vi "PololuTicSendCommand.vi"(4 "Type":string(combo), 5 "Address":u16=16384 max=16384, 6 "Register":u8 format="%02x", 7 "Port Name":refnum<visa-resource-name>, 8 "errorIn":errorcluster, 10 "Argument":i32, 11 "PololuCommand":T2="FullScaleRatingSLPM") -> (0 "errorOut":errorcluster, 1 "LSB                                       MSB":bool[](array[boolean]) caption="Booleans", 2 "ReadValue":i64, 3 "Response":string)   [LabVIEW 2021]
uses:
  PololuCommand.ctl
  TicReplyStyle.ctl
panel:
  in  "Timeout/ms":u32=2000
  in  "ReplyType [7-bit]":T1=enum."7-bit"
  # "[16384=Unaddressed/Global]"
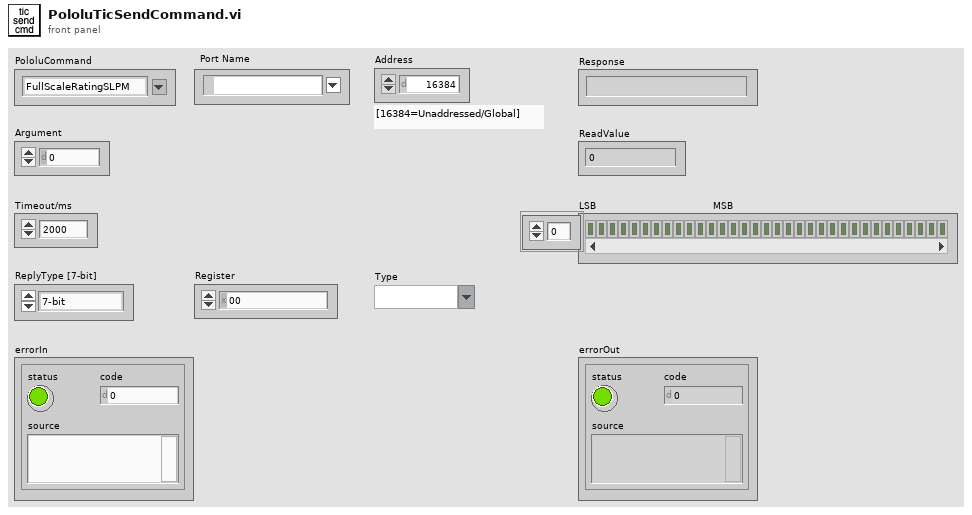
[diagram p1: front panel]
types:
  T1 = typedef "TicReplyStyle.ctl" = enum16{"8-bit", "7-bit"}
  T2 = typedef "PololuCommand.ctl" = string
  T3 = typedef "PololuCommandDescriptor.ctl" = cluster{"PololuCommand":string, "Mnemonic":string, "CommandType":T4, "Min":i32, "Max":i32}
  T4 = typedef "TicCommandType.ctl" = enum16{"Command", "7-bitWrite", "32-bitWrite", "BlockRead"}
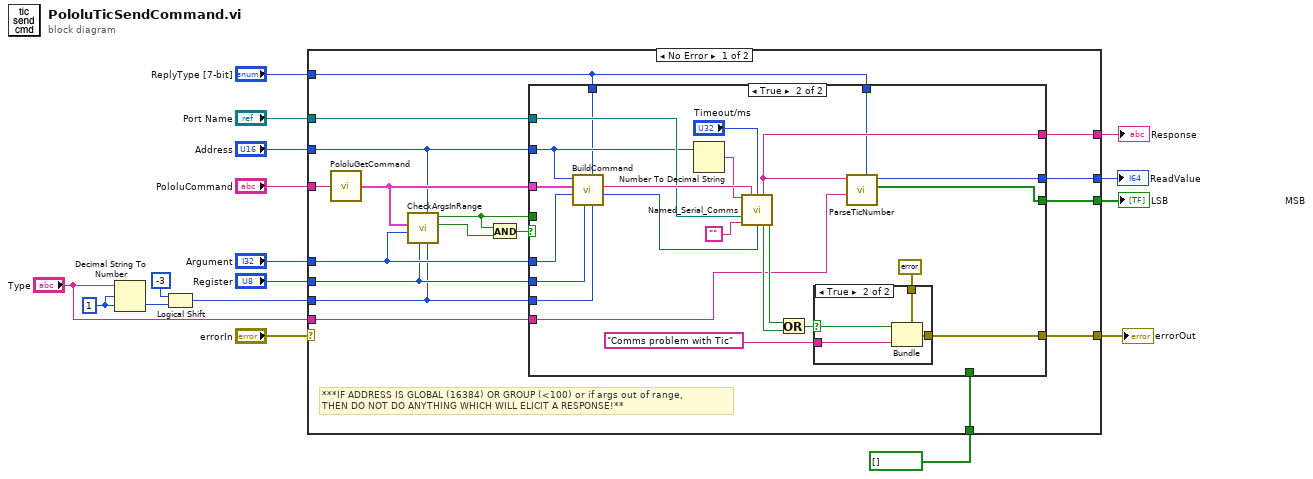
[diagram p0: block diagram]
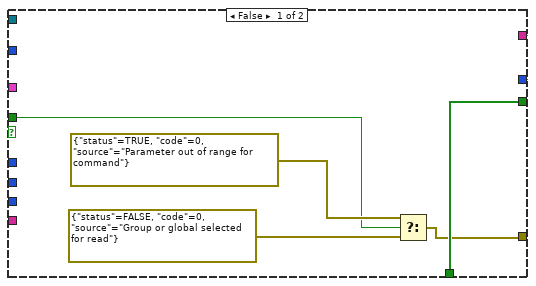
[diagram p2: hidden frame]
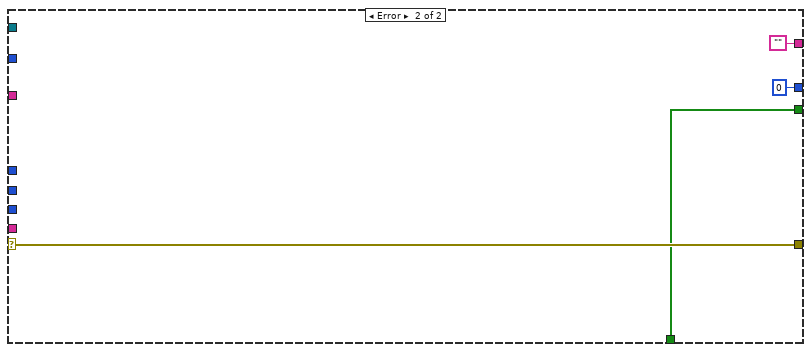
[diagram p4: hidden frame]
diagram:
  w4 = u8 1 ("offset")
  n1 = Decimal String To Number(string="Type", offset=w4, default (0L)=w4) -> (number=w7:u8)  [unwired: 1 out]
  n2 = Logical Shift(y=i16 -3, x=w7) -> (x << y=w5:u8)
  n3 = case shown="No Error" "errorIn" {
    selector: "errorIn" -> [_ w73]
    tunnel: "PololuCommand" -> [w34 _]
    tunnel: [w33 "" ("Read")] -> w16
    tunnel: [w32 i64 0 ("Value")] -> w15
    tunnel: [w31 w71] -> w14
    tunnel: [w30 w73] -> w13
    tunnel: "Argument" -> [w28 _]
    tunnel: "Register" -> [w27 _]
    tunnel: w5 -> [w26 _]
    tunnel: "Address" -> [w21 _]
    tunnel: "Port Name" -> [w25 _]
    tunnel: "Type" -> [w24 _]
    tunnel: "ReplyType [7-bit]" -> [w23 _]
    tunnel: bool[] [] ("Boolean array") -> [w22 w71]
    frame No Error {
      # "***IF ADDRESS IS GLOBAL (16384) OR GROUP (<100) or if args out of range,\nTHEN DO NOT DO ANYTHING WHICH WILL ELICIT A RESPONSE!**"
      n4 = call "PololuGetCommand.vi"("PololuCommand"=w34) -> ("CommandDescriptor"=w29:T3)  [unwired: 3 in, 1 out]
      n5 = call "CheckArgsInRange.vi"("ReadLength (bytes)"=w26, "Address"=w21, "Register"=w27, "Argument"=w28, "CommandDescriptor in"=w29) -> ("In Range?"=w19:bool, "Not Group/Global?"=w20:bool)  [unwired: 5 in]
      n6 = And(x=w20, y=w19) -> (x .and. y?=w18:bool)
      n7 = case shown="True" w18 {
        tunnel: w27 -> [_ w56]
        tunnel: w29 -> [_ w60]
        tunnel: ["" w61] -> w33
        tunnel: [0 ("Value") w64] -> w32
        tunnel: w26 -> [_ w46]
        tunnel: w22 -> [w40 _]
        tunnel: [w40 w63] -> w31
        tunnel: w28 -> [_ w57]
        tunnel: [w36 w54] -> w30
        tunnel: w21 -> [_ w48]
        tunnel: w25 -> [_ w55]
        tunnel: w24 -> [_ w43]
        tunnel: w23 -> [_ w45]
        tunnel: w23 -> [_ w44]
        tunnel: w20 -> [w35 _]
        frame False {
          n8 = Select(t=errorcluster {"status"=TRUE, "code"=0, "source"="Parameter out of range for command"} ("error out"), s=w35, f=errorcluster {"status"=FALSE, "code"=0, "source"="Group or global selected for read"} ("error out")) -> (s? t:f=w36:errorcluster)
        }
        frame True {
          n9 = call "BuildCommand.vi"("ReadLength (bytes) in"=w46, "ReplyType [7-bit]"=w45, "Register"=w56, "Argument"=w57, "CommandDescriptor"=w60, "Address"=w48) -> ("ReadLength (bytes) out"=w58:u8, "AssembledCommand"=w59:string)  [unwired: 4 in]
          n10 = Number To Decimal String(number=w48) -> (decimal integer string=w47:string)  [unwired: 1 in]
          n11 = call "Named_Serial_Comms.vi"("Channel Name"=w47, "Write"=w59, "Timeout/ms"="Timeout/ms", "Port Name"=w55, "Term Grep"="", "Terminate Count"=w58) -> ("Read"=w61:string, "Timed out"=w51:bool, "Serial Error"=w50:bool)  [unwired: 5 in, 2 out]
          n12 = Or(x=w50, y=w51) -> (x .or. y?=w52:bool)
          n13 = case shown="True" w52 {
            selector: w52 -> [_ w67]
            tunnel: [w65 w69] -> w54
            tunnel: errorcluster {"status"=FALSE, "code"=0, "source"=""} ("errorIn") -> [w65 w68]
            tunnel: "Comms problem with Tic" -> [_ w66]
            frame False {
            }
            frame True {
              n14 = Bundle(cluster=w68, "status"=w67, "source"=w66) -> (w69:errorcluster)  [unwired: 1 in]
            }
          }
          n15 = call "ParseTicNumber.vi"("ReplyType [7-bit]"=w44, "Type"=w43, "Read"=w61) -> ("LSB                   MSB"=w63:bool[], "Value"=w64:i64)  [unwired: 7 in]
        }
      }
    }
    frame Error {
    }
  }
  "Response" <- w16
  "ReadValue" <- w15
  "LSB                                       MSB" <- w14
  "errorOut" <- w13
